vi "FixPath.vi"(11 "path string":string) -> (3 "path":path)   [LabVIEW 2015]
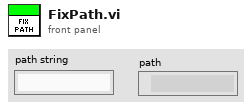
[diagram p1: front panel]
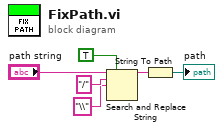
[diagram p0: block diagram]
diagram:
  n1 = Search and Replace String(replace all?=TRUE ("replace all? (F)"), input string="path string", search string="/", replace string="\\" ("search string")) -> (result string=w2:string)  [unwired: 4 in, 3 out]
  n2 = String To Path(string=w2) -> (path=→"path":path)
